vi "String Functions 3b.vi"() -> ()   [LabVIEW 2020]
panel:
  out "Lower Case Output":string
  out "Upper Case Output":string
  in  "String Input":string
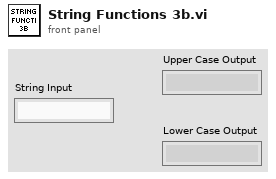
[diagram p1: front panel]
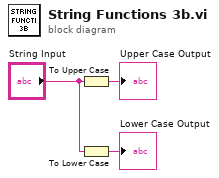
[diagram p0: block diagram]
diagram:
  n1 = To Upper Case(1:"String Input") -> (0:→"Upper Case Output":string)
  n2 = To Lower Case(string="String Input") -> (all lower case string=→"Lower Case Output":string)
